vi "Send Nested Actor Message.vi"(8 "error in (no error)":errorcluster, 9 "Message":string, 10 "Actor Name":string, 11 "Calling Actor in":refnum<class "Calling Actor.lvclass">) -> (0 "error out":errorcluster, 3 "Calling Actor out":refnum<class "Calling Actor.lvclass">)   [LabVIEW 2019, in "Calling Actor.lvlib" / "Calling Actor.lvclass"]
uses:
  Calling Actor.lvclass
  Calling Actor.lvclass/Calling Actor.ctl
  Nested Actor Messages/Update Message Indicator Msg/Update Message Indicator Msg.lvclass/Update Message Indicator Msg.ctl
  <vilib>/ActorFramework/Message Enqueuer/Message Enqueuer.lvclass/Message Enqueuer.ctl
  <vilib>/ActorFramework/Message Enqueuer/Enqueue.vi
  Nested Actor Messages/Update Message Indicator Msg/Update Message Indicator Msg.lvclass
  C:/Program Files (x86)/National Instruments/LabVIEW 2019/vi.lib/ActorFramework/Message/Message.lvclass
  <vilib>/ActorFramework/Message Priority Queue/Priority Enqueue.vi
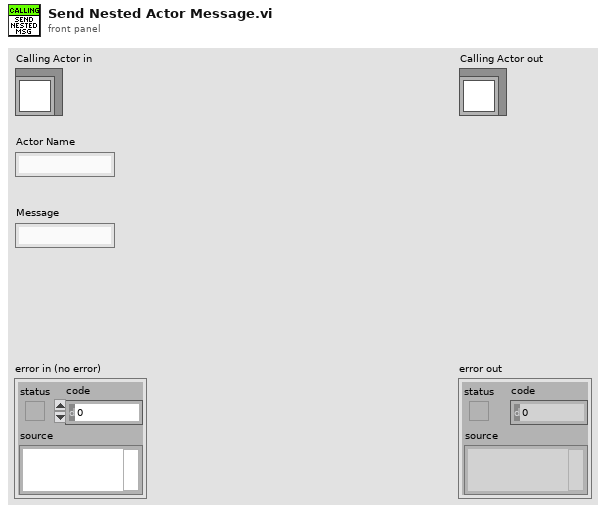
[diagram p1: front panel]
types:
  T1 = map{string, refnum<class "Message Enqueuer.lvclass">}
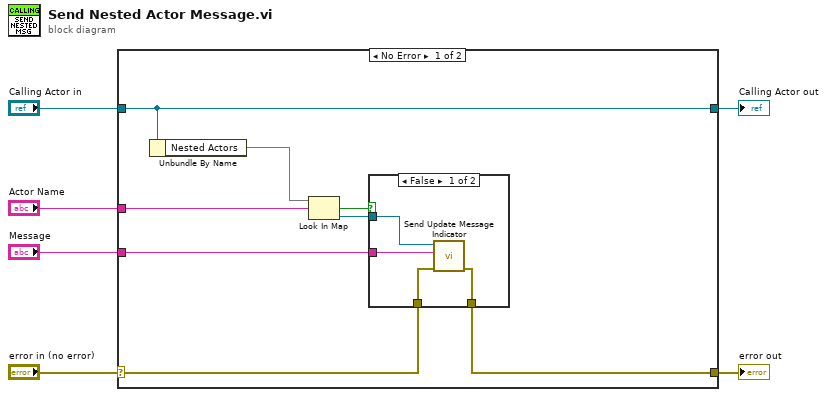
[diagram p0: block diagram]
diagram:
  n1 = case shown="No Error" "error in (no error)" {
    selector: "error in (no error)" -> [w13 w21]
    tunnel: [w12 w21] -> w5
    tunnel: [w11 w20] -> w3
    tunnel: "Calling Actor in" -> [w11 w20]
    tunnel: "Actor Name" -> [w9 _]
    tunnel: "Message" -> [w14 _]
    frame No Error {
      n2 = Unbundle By Name(w11) -> ("Nested Actors"=w10:T1)
      n3 = Look In Map(map=w10, key=w9) -> (key not found?=w7:bool, value=w8:refnum<class "Message Enqueuer.lvclass">)  [unwired: 1 in]
      n4 = case shown="False" w7 {
        tunnel: w14 -> [w18 _]
        tunnel: w13 -> [w17 w19]
        tunnel: [w16 w19] -> w12
        tunnel: w8 -> [w15 _]
        frame False {
          n5 = call "Send Update Message Indicator.vi"("error in (no error)"=w17, "Message From Caller"=w18, "Message Enqueuer"=w15) -> ("error out"=w16:errorcluster)  [unwired: 7 in, 1 out]
        }
        frame True {
        }
      }
    }
    frame Error {
    }
  }
  "error out" <- w5
  "Calling Actor out" <- w3
